vi "GenerateFolderDiagram.vi"(8 "error in":errorcluster, 10 "Numeric":i32, 11 "created path in":path) -> (0 "error out":errorcluster, 3 "created path out":path)   [LabVIEW 2017]
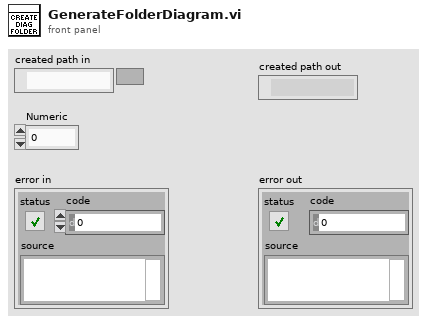
[diagram p1: front panel]
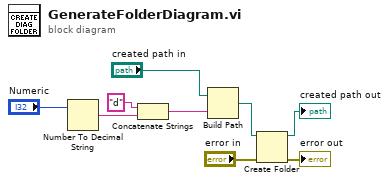
[diagram p0: block diagram]
diagram:
  n1 = Number To Decimal String(number="Numeric") -> (decimal integer string=w7:string)  [unwired: 1 in]
  n2 = Concatenate Strings("d" ("string"), w7) -> (w3:string)
  n3 = Build Path(base path="created path in", name or relative path=w3) -> (appended path=w1:path)
  n4 = Create Folder(path (use dialog)=w1, error in="error in") -> (created path=→"created path out":path, error out=→"error out":errorcluster)  [unwired: 1 in, 1 out]
